vi "Write_Path_to_Command_List.vi"(0 "LastCmdNumb":i32=64, 4 "CmdNumb":i32=62, 5 "WayPoints":T1[](array[typedef])=[{"x"=15.0, "y"=105.0, "angle"=0.0}, {"x"=35.0, "y"=105.0, "angle"=0.0}, {"x"=210.0, "y"=32.0, "angle"=0.0}, {"x"=230.0, "y"=32.0, "angle"=0.0}], 6 "FirstCmdNumb":i32=60, 7 "Include Step":bool=TRUE, 8 "Wheel_Ctrl_Elements":T2 {"Wheel_Ctrl_Elements"."D Time" format="%13.3f"; "Wheel_Ctrl_Elements"."Angle" format="%13.3f"; "Wheel_Ctrl_Elements"."R dist" format="%13.3f"; "Wheel_Ctrl_Elements"."L dist" format="%13.3f"; "Wheel_Ctrl_Elements"."R spd" format="%13.3f"; "Wheel_Ctrl_Elements"."L spd" format="%13.3f"; "Wheel_Ctrl_Elements"."T Time" format="%13.3f"}, 9 "Comment":string, 10 "starting step":i32, 11 "Cmd List File":path) -> ()   [LabVIEW 2018]
uses:
  Pathfinder-Lib/VIs/Wheel_Ctrl_Path.ctl
  Pathfinder-Lib/VIs/Wheel_Ctrl_Path_Element.ctl
  Pathfinder-Lib/VIs/Waypoint.ctl
  Pathfinder-Lib/Pathfinder.lvlib
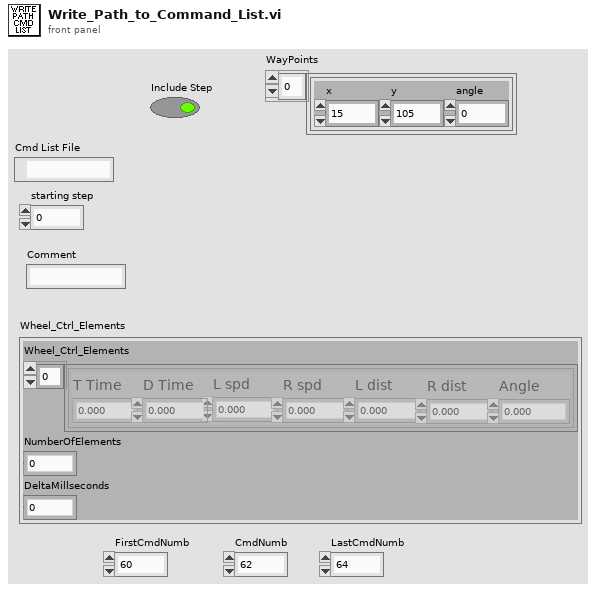
[diagram p1: front panel]
types:
  T1 = typedef "Pathfinder.lvlib/Waypoint.ctl" = cluster{"x":dbl, "y":dbl, "angle":dbl}
  T2 = typedef "Pathfinder.lvlib/Wheel_Ctrl_Path.ctl" = cluster{"Wheel_Ctrl_Elements":T3[], "NumberOfElements":u32, "DeltaMillseconds":i32}
  T3 = typedef "Pathfinder.lvlib/Wheel_Ctrl_Path_Element.ctl" = cluster{"T Time":dbl, "L spd":dbl, "R spd":dbl, "L dist":dbl, "R dist":dbl, "Angle":dbl, "D Time":dbl}
  T4 = enum16{"open", "replace", "create", "open or create", "replace or create", "replace or create with confirmation"}
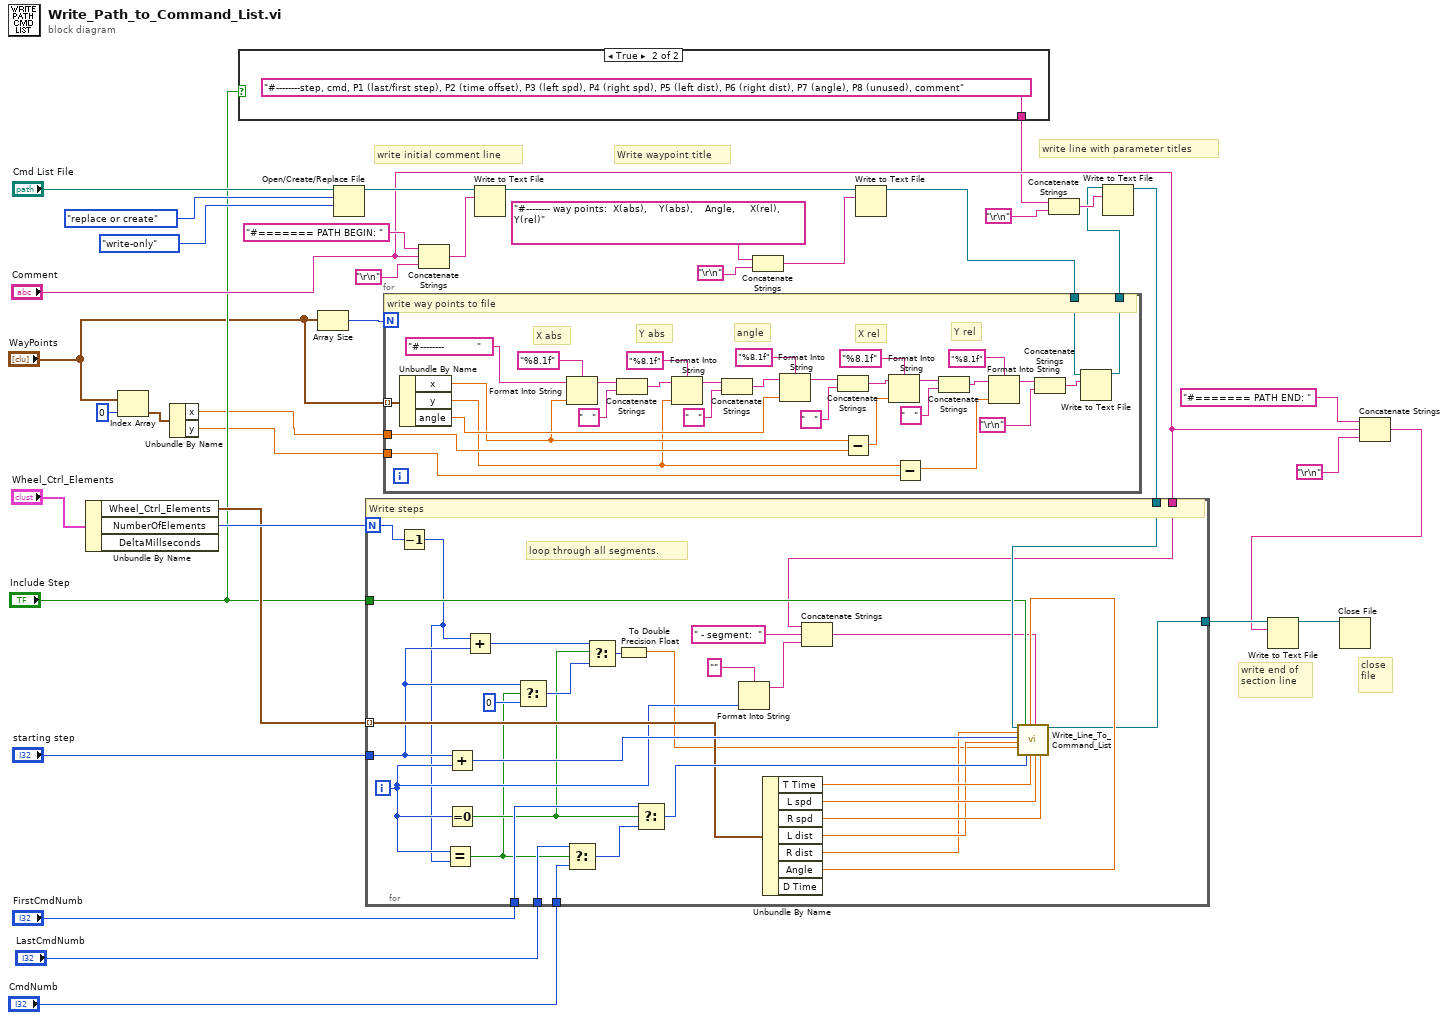
[diagram p0: block diagram]
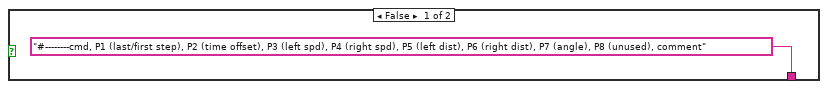
[diagram p2: hidden frame]
diagram:
  # "Write waypoint title"
  # "close\nfile"
  # "write end of\nsection line"
  # "write line with parameter titles"
  # "write initial comment line"
  n1 = Unbundle By Name("Wheel_Ctrl_Elements") -> ("Wheel_Ctrl_Elements"=w35:T3[], "NumberOfElements"=w36:u32)  [unwired: 1 out]
  n2 = Index Array(array="WayPoints", index=0) -> (element=w11:T1)
  n3 = Unbundle By Name(w11) -> ("x"=w6:dbl, "y"=w5:dbl)
  n4 = case shown="True" "Include Step" {
    tunnel: ["#--------cmd, P1 (last/first step), P2 (time offset), P3 (left spd), P4 (right spd), P5 (left dist), P6 (right dist), P7 (angle), P8 (unused), comment" ("string") "#--------step, cmd, P1 (last/first step), P2 (time offset), P3 (left spd), P4 (right spd), P5 (left dist), P6 (right dist), P7 (angle), P8 (unused), comment" ("string")] -> w14
    frame False {
    }
    frame True {
    }
  }
  n5 = Array Size(array="WayPoints") -> (size(s)=w10:i32)
  n6 = Open/Create/Replace File(file path (use dialog)="Cmd List File", operation (0:open)=T4."replace or create", access (0:read/write)=enum16{"read/write", "read-only", "write-only"}."write-only") -> (refnum out=w30:refnum<file>)  [unwired: 3 in, 2 out]
  n7 = Concatenate Strings("#======= PATH BEGIN: " ("string"), "Comment", "\r\n") -> (w27:string)
  n8 = Write to Text File(file (use dialog)=w30, text=w27) -> (refnum out=w8:refnum<file>)  [unwired: 2 in, 2 out]
  n9 = Concatenate Strings("#-------- way points:  X(abs),    Y(abs),    Angle,     X(rel),    Y(rel)" ("string"), "\r\n") -> (w3:string)
  n10 = Write to Text File(file (use dialog)=w8, text=w3) -> (refnum out=w2:refnum<file>)  [unwired: 2 in, 2 out]
  n11 = for {
    N: w10 -> [_]
    tunnel: "WayPoints" -> [w60] mode=indexing
    tunnel: w6 -> [w59]
    tunnel: w5 -> [w58]
    tunnel: w2 -> [w55]
    tunnel: [w54] -> w1
    # "Y rel"
    # "X rel"
    # "angle"
    # "Y abs"
    # "X abs"
    # "write way points to file"
    n12 = Unbundle By Name(w60) -> ("x"=w43:dbl, "y"=w42:dbl, "angle"=w57:dbl)
    n13 = Format Into String(format string="%8.1f", initial string="#--------           " ("string"), w43) -> (resulting string=w70:string)  [unwired: 1 in, 1 out]
    n14 = Concatenate Strings(w70, "   " ("string")) -> (w68:string)
    n15 = Format Into String(format string="%8.1f", initial string=w68, w42) -> (resulting string=w69:string)  [unwired: 1 in, 1 out]
    n16 = Concatenate Strings(w69, "   " ("string")) -> (w67:string)
    n17 = Format Into String(format string="%8.1f", initial string=w67, w57) -> (resulting string=w56:string)  [unwired: 1 in, 1 out]
    n18 = Concatenate Strings(w56, "   " ("string")) -> (w50:string)
    n19 = Subtract(x=w43, y=w59) -> (x-y=w41:dbl)
    n20 = Format Into String(format string="%8.1f", initial string=w50, w41) -> (resulting string=w53:string)  [unwired: 1 in, 1 out]
    n21 = Subtract(x=w42, y=w58) -> (x-y=w40:dbl)
    n22 = Concatenate Strings(w53, "   " ("string")) -> (w49:string)
    n23 = Format Into String(format string="%8.1f", initial string=w49, w40) -> (resulting string=w45:string)  [unwired: 1 in, 1 out]
    n24 = Concatenate Strings(w45, "\r\n") -> (w44:string)
    n25 = Write to Text File(file (use dialog)=w55, text=w44) -> (refnum out=w54:refnum<file>)  [unwired: 2 in, 2 out]
  }
  n26 = Concatenate Strings(w14, "\r\n") -> (w26:string)
  n27 = Write to Text File(file (use dialog)=w1, text=w26) -> (refnum out=w29:refnum<file>)  [unwired: 2 in, 2 out]
  n28 = for {
    N: w36 -> [w90]
    tunnel: w35 -> [w99] mode=indexing
    tunnel: "starting step" -> [w78]
    tunnel: [w92] -> w18
    tunnel: w29 -> [w91]
    tunnel: "CmdNumb" -> [w89]
    tunnel: "LastCmdNumb" -> [w88]
    tunnel: "FirstCmdNumb" -> [w87]
    tunnel: "Include Step" -> [w86]
    tunnel: "Comment" -> [w81]
    i -> [w82]
    # "loop through all segments."
    # "Write steps"
    n29 = Decrement(x=w90) -> (x-1=w77:i32)
    n30 = Equal?(x=w82, y=w77) -> (x = y?=w71:bool)
    n31 = Add(x=w78, y=w82) -> (x+y=w102:i32)
    n32 = Equal To 0?(x=w82) -> (x = 0?=w72:bool)
    n33 = Add(x=w77, y=w78) -> (x+y=w76:i32)
    n34 = Select(t=w78, s=w71, f=0) -> (s? t:f=w79:i32)
    n35 = Select(t=w88, s=w71, f=w89) -> (s? t:f=w101:i32)
    n36 = Select(t=w76, s=w72, f=w79) -> (s? t:f=w74:i32)
    n37 = To Double Precision Float(number=w74) -> (double precision float=w73:dbl)
    n38 = Select(t=w87, s=w72, f=w101) -> (s? t:f=w100:i32)
    n39 = Format Into String(format string="", w82) -> (resulting string=w84:string)  [unwired: 2 in, 1 out]
    n40 = Unbundle By Name(w99) -> ("T Time"=w98:dbl, "L spd"=w97:dbl, "R spd"=w96:dbl, "L dist"=w95:dbl, "R dist"=w94:dbl, "Angle"=w93:dbl)  [unwired: 1 out]
    n41 = Concatenate Strings(w81, " - segment:  " ("string"), w84) -> (w80:string)
    n42 = call "Write_Line_To_Command_List.vi"("Byte Stream File in"=w91, "P6"=w94, "Step"=w102, "P5"=w95, "P1"=w73, "Include Step"=w86, "CmdNumb"=w100, "P7"=w93, "P2"=w98, "Comment"=w80, "P3"=w97, "P4"=w96) -> ("Byte Stream File out"=w92:refnum<file>)  [unwired: 7 in]
  }
  n43 = Concatenate Strings("#======= PATH END: " ("string"), "Comment", "\r\n") -> (w16:string)
  n44 = Write to Text File(file (use dialog)=w18, text=w16) -> (refnum out=w17:refnum<file>)  [unwired: 2 in, 2 out]
  n45 = Close File(refnum=w17) -> ()  [unwired: 1 in, 2 out]
